vi "Test Relative Path.vi"(4 "File Name":string, 5 "File Path Control in":path) -> (2 "File Path Control Out":path)   [LabVIEW 2015]
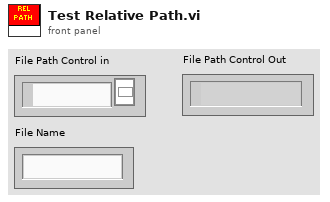
[diagram p1: front panel]
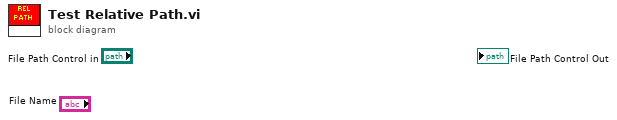
[diagram p0: block diagram]
diagram:
